vi "Get Unit Conversion Per Volt.vi"(0 "Accel Sensitivity (mV/ms-2)":dbl, 11 "error in (no error)":errorcluster) -> (8 "mV/(in/s2)":dbl, 10 "mV/(m/s2)":dbl, 15 "error out":errorcluster)   [LabVIEW 2014, in "RT - Analysis.lvlib"]
doc: "Calculates the value for conversion between inches/sec^2 and Volts\nusing channel name and Range/Span values"
uses:
  RT - Analysis.lvlib
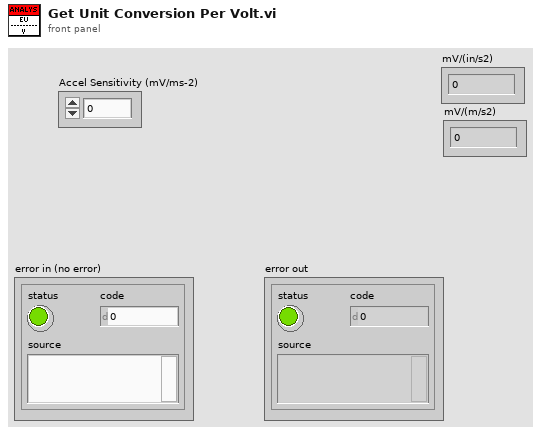
[diagram p1: front panel]
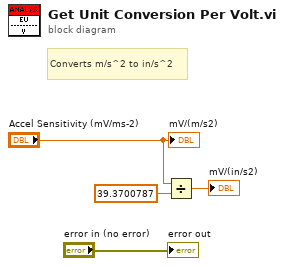
[diagram p0: block diagram]
diagram:
  # "Converts m/s^2 to in/s^2"
  n1 = Divide(x="Accel Sensitivity (mV/ms-2)", y=39.3700787) -> (x/y=→"mV/(in/s2)":dbl)
  "error out" <- "error in (no error)"
  "mV/(m/s2)" <- "Accel Sensitivity (mV/ms-2)"
